vi "PCO_GetNumberOfImagesInSegment.vi"(8 "error in (no error)":errorcluster, 11 "Handle":u64) -> (0 "error out":errorcluster, 3 "Handle Out":u64, 5 "return type":u32 format="%x")   [LabVIEW 2011]
uses:
  SC2_Cam64.dll
panel:
  out "dwMaxImageCnt":i32
  out "dwValidImageCnt":i32
  in  "wSegment 1..4":u16=1
  # "fifo:lost Images?"
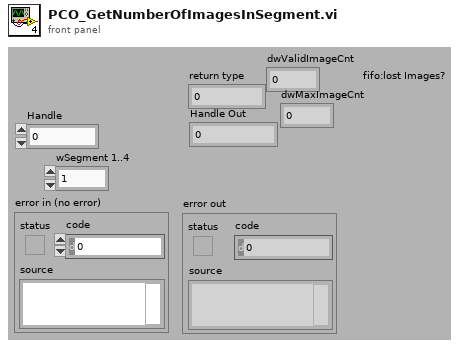
[diagram p1: front panel]
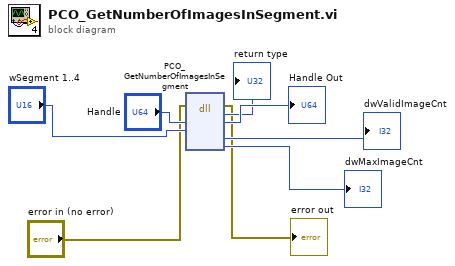
[diagram p0: block diagram]
diagram:
  n1 = dll-call lib="SC2_Cam*.*" fn="PCO_GetNumberOfImagesInSegment"(error in="error in (no error)", "Handle"="Handle", "wSegment"="wSegment 1..4") -> (error out=→"error out":errorcluster, "return type"=→"return type":u32, "Handle"=→"Handle Out":u64, "dwValidImageCnt"=→"dwValidImageCnt":i32, "dwMaxImageCnt"=→"dwMaxImageCnt":i32)  [unwired: 3 in, 3 out]
